vi "host_as ETH hub.vi"() -> ()   [LabVIEW 2021]
uses:
  <vilib>/userdefined/High Color/nirio_resource_hc.ctl
  CTL/states.ctl
  classes/P2P from the network/P2P from the network.lvclass
  CTL/user config.ctl
panel:
  out "error out":errorcluster
  out "Enum":T1
  in  "update and start":bool
  in  "num of PDW on fifo before starting secenario":u32
  in  "P2P sample rate":dbl format="%#_6pHz"
  in  "center frequency (Hz)":dbl format="%#_6pHz"
  in  "RF max power":dbl format="%#_gdBm"
  out "pulse transmitted":u32
  out "num of pulses sent to the FPGA":u32
  in  "devicess":T2[](array[typedef])=["IF_transceiver_0", "IF_transceiver_1", "IF_transceiver_2"]
  in  "receiver port":u16=8800
  in  "vst_device":refnum<k15>[](array[refnum])=["VST_5840"]
  out "secnario elapest 2":dbl
  out "dds free":bool[][](array[boolean])=[[TRUE, FALSE, FALSE, FALSE, FALSE, FALSE], [TRUE, FALSE, FALSE, FALSE, FALSE, FALSE], [TRUE, FALSE, FALSE, FALSE, FALSE, FALSE], [TRUE, FALSE, FALSE, FALSE, FALSE, FALSE], [TRUE, FALSE, FALSE, FALSE, FALSE, FALSE], [TRUE, FALSE, FALSE, FALSE, FALSE, FALSE], [TRUE, FALSE, FALSE, FALSE, FALSE, FALSE], [TRUE, FALSE, FALSE, FALSE, FALSE, FALSE], [TRUE, FALSE, FALSE, FALSE, FALSE, FALSE], [TRUE, TRUE, TRUE, TRUE, TRUE, TRUE], [TRUE, TRUE, TRUE, TRUE, TRUE, TRUE], [TRUE, TRUE, TRUE, TRUE, TRUE, TRUE], [TRUE, TRUE, TRUE, TRUE, TRUE, TRUE], [TRUE, TRUE, TRUE, TRUE, TRUE, TRUE], [TRUE, TRUE, TRUE, TRUE, TRUE, TRUE], [TRUE, TRUE, TRUE, TRUE, TRUE, TRUE]]
  # "HW"
  # "RF setup"
  # "Tx state"
  # "Control"
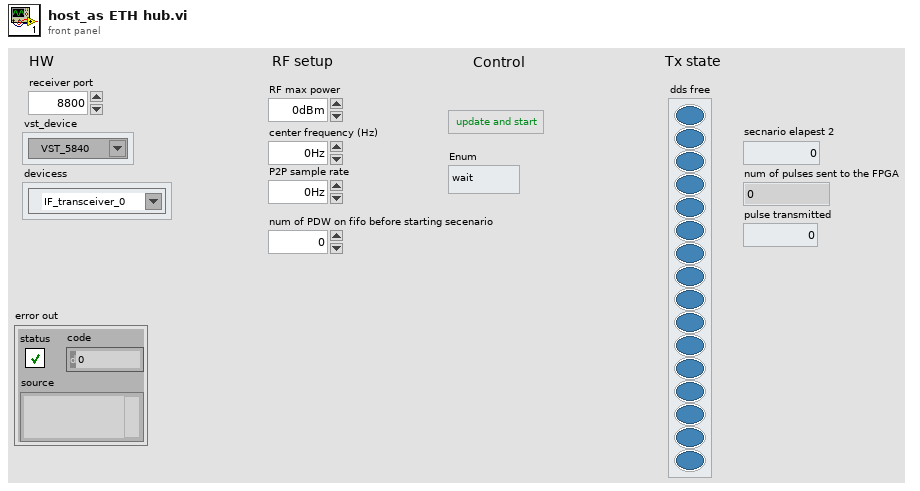
[diagram p1: front panel]
types:
  T1 = typedef "states.ctl" = enum16{"wait", "update config", "ini for transmit", "prime the fifo", "sync and trig", "transmit", "close sesion", "close program", "import secenario from csv", "generate secenario", "refresh file display", "export file", "reset sesion"}
  T2 = typedef "nirio_resource_hc.ctl" = tag
  T3 = typedef "user config.ctl" = cluster{"vst_device":refnum<k15>[], "RF gain ":dbl, "buffer size":u32, "center frequency (Hz) ":dbl, "P2P sample rate":dbl, "mode":enum16{"USRP - 180MHz", "5785 - 2*180MHz", "5785 - 3.2GHz", "P2P - VST"}, "devicess":T2[], "gen for df":bool, "Rx settings":cluster{"min PW         ":dbl, "max gap        ":dbl, "detection bar":dbl, "peak detect                        ":bool}, "IQ file":path}
  T4 = cluster{"fpga clock":dbl, "pulse transmitted":u32, "dds free":bool[][]}
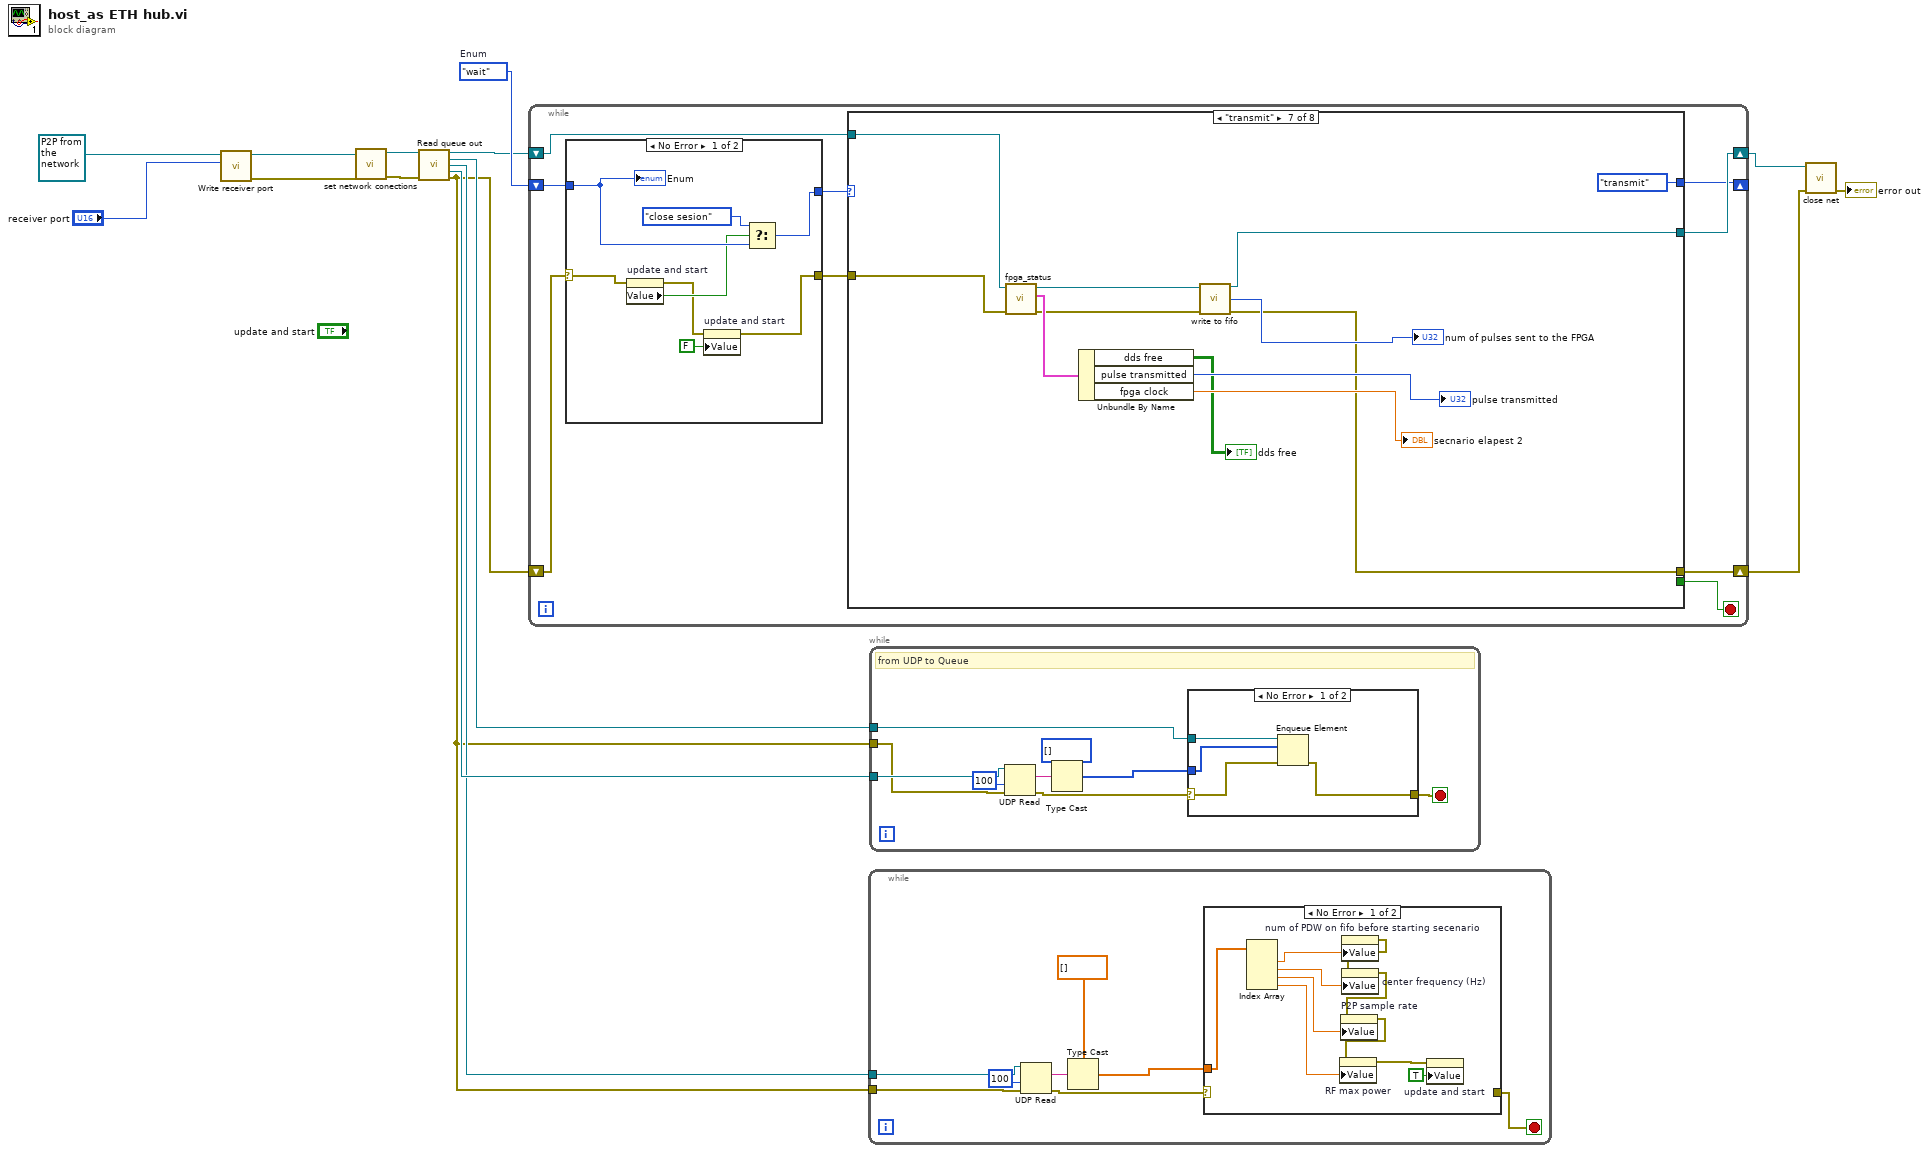
[diagram p0: block diagram]
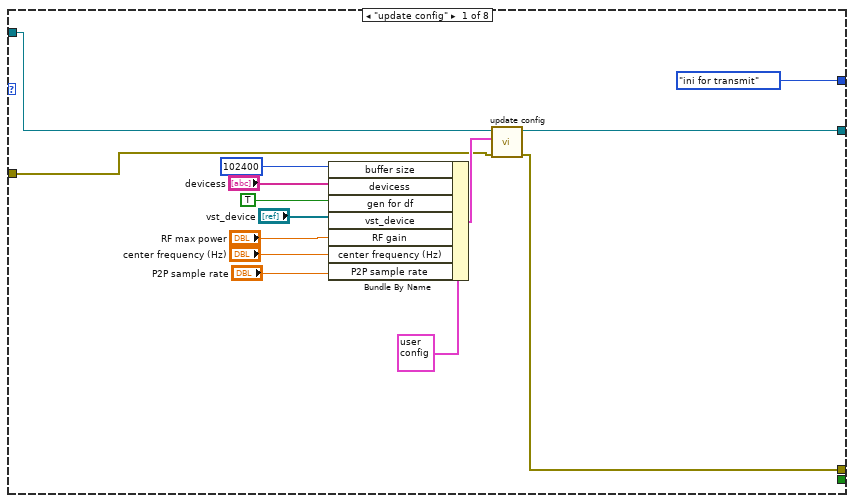
[diagram p2: hidden frame]
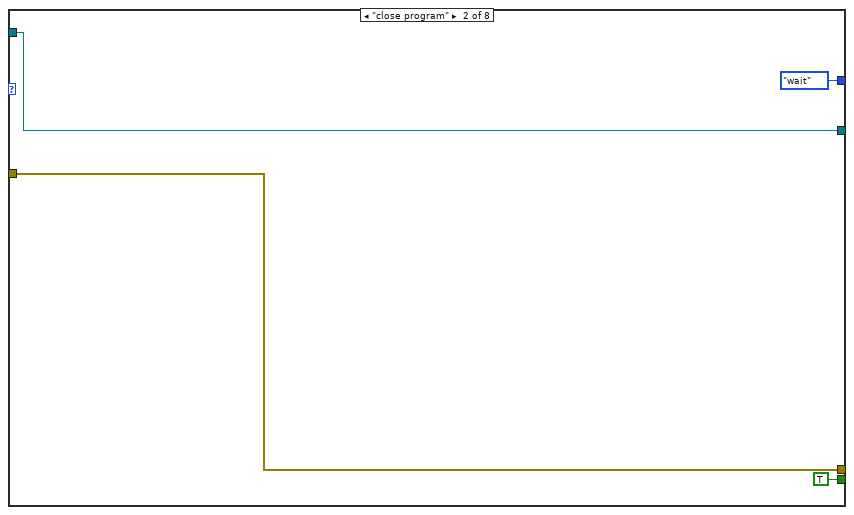
[diagram p3: hidden frame]
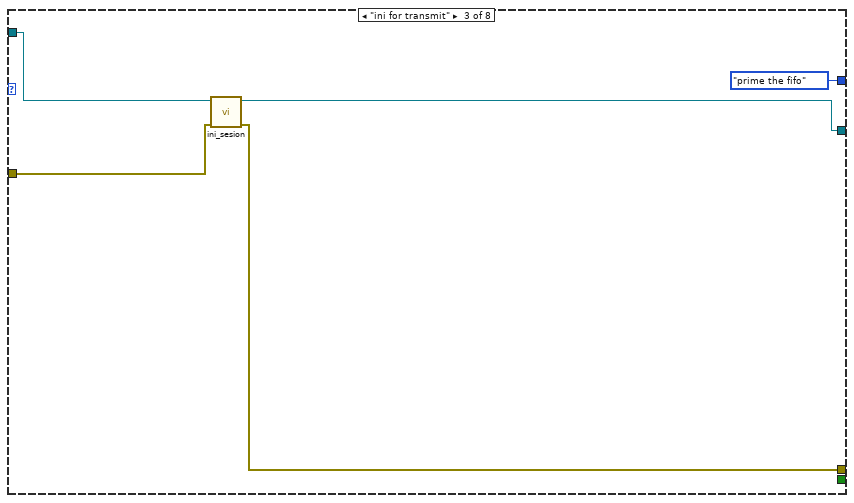
[diagram p4: hidden frame]
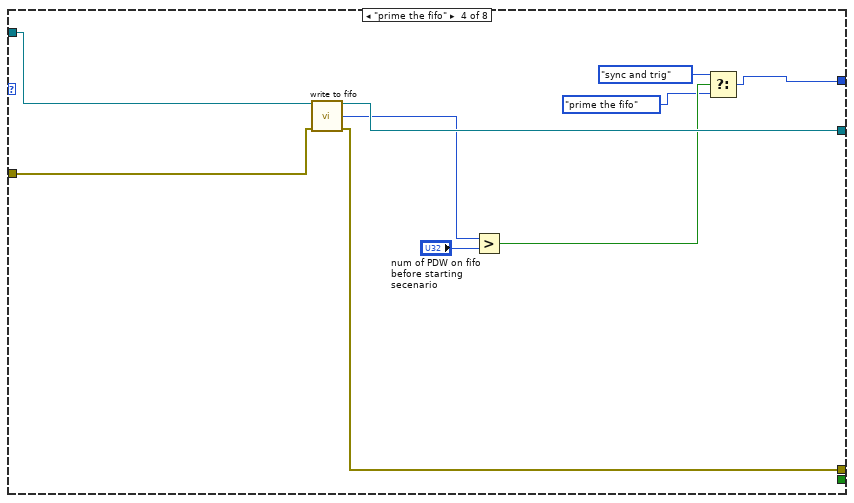
[diagram p5: hidden frame]
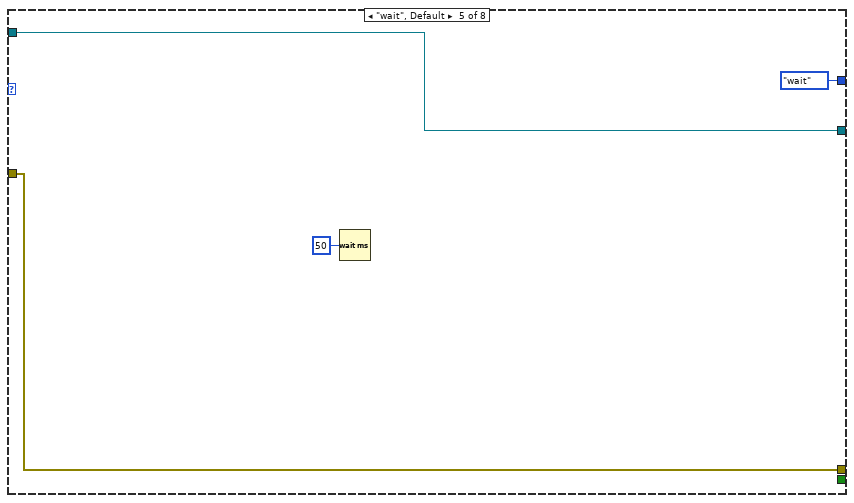
[diagram p6: hidden frame]
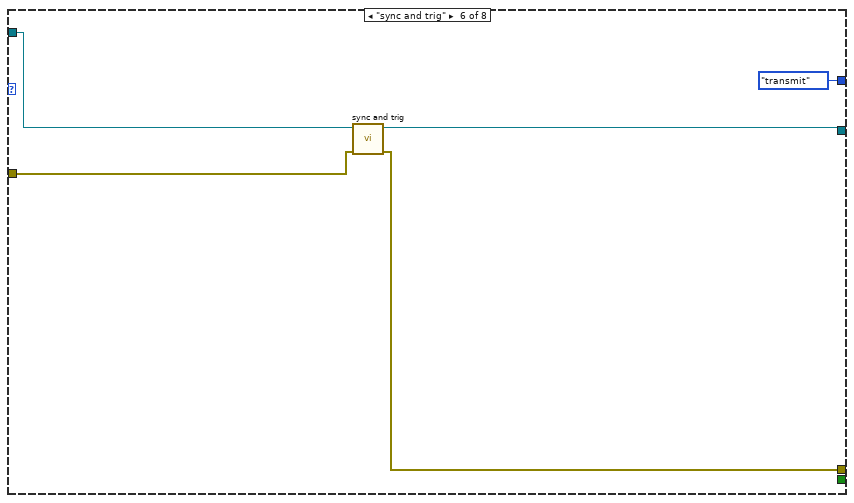
[diagram p7: hidden frame]
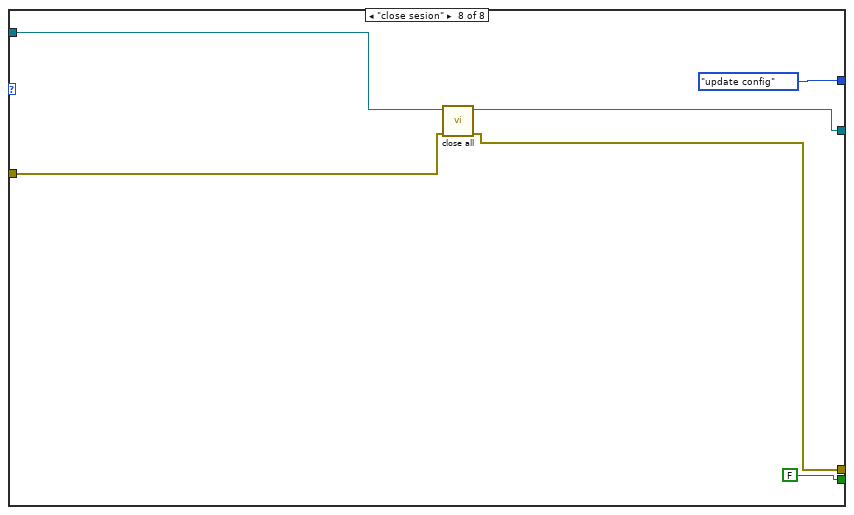
[diagram p8: hidden frame]
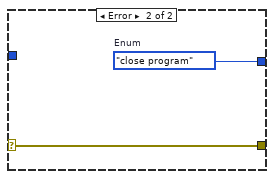
[diagram p9: hidden frame]
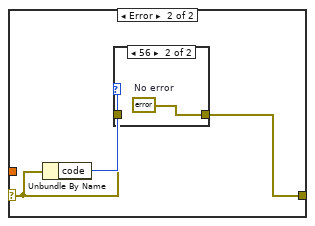
[diagram p10: hidden frame]
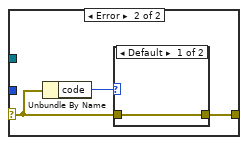
[diagram p12: hidden frame]
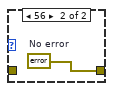
[diagram p13: hidden frame]
diagram:
  w8 = states."wait"  # Enum
  n1 = call-dynamic "Write receiver port.vi"("receiver port"="receiver port", "P2P from the network in"=refnum<class "P2P from the network.lvclass"> refnum ("P2P from the network.lvclass")) -> ("error out"=w10:errorcluster, "P2P from the network out"=w11:refnum<class "P2P from the network.lvclass">)  [unwired: 8 in]
  n2 = call-dynamic "set network conections.vi"("error in (no error)"=w10, "P2P from the network in"=w11) -> ("error out"=w6:errorcluster, "P2P from the network out"=w7:refnum<class "P2P from the network.lvclass">)  [unwired: 8 in]
  n3 = call-dynamic "Read queue out.vi"("P2P from the network in"=w7, "error in (no error)"=w6) -> ("P2P from the network out"=w4:refnum<class "P2P from the network.lvclass">, "queue out"=w14:refnum<queue>, "connection ID control port"=w9:refnum<k16>, "connection ID PDW"=w15:refnum<k16>, "error out"=w5:errorcluster)  [unwired: 9 in]
  n4 = while {
    shift-right: [w16] -> _
    shift-left: w8 -> [w23]
    shift-right: [w18] -> w2
    shift-left: w5 -> [w24]
    shift-right: [w19] -> w3
    shift-left: w4 -> [w21]
    stop <- w17 stop-if-true
    n5 = case shown="No Error" w24 {
      selector: w24 -> [w86 w93]
      tunnel: w23 -> [w92 _]
      tunnel: [w91 w94] -> w22
      tunnel: [w85 w93] -> w20
      frame No Error {
        n6 = property on="update and start" class="Bool (strict)"(error in=w86) -> (error out=w88:errorcluster, "Value"=w89:bool)  [unwired: 1 in, 1 out]
        n7 = property on="update and start" class="Bool (strict)"(error in=w88, "Value"=FALSE ("update and start")) -> (error out=w85:errorcluster)  [unwired: 1 in, 1 out]
        n8 = Select(t=states."close sesion", s=w89, f=w92) -> (s? t:f=w91:T1)
        "Enum" <- w92
      }
      frame Error {
        w94 = states."close program"  # Enum
      }
    }
    n9 = case shown="\"transmit\"" w22 {
      tunnel: w21 -> [w28 w39 w47 w57 w60 w66 w70 w82]
      tunnel: w20 -> [w29 w41 w46 w55 w59 w64 w71 w80]
      tunnel: [w27 w39 w45 w56 w60 w65 w69 w81] -> w19
      tunnel: [states."ini for transmit" ("Enum") states."wait" ("Enum") states."prime the fifo" ("Enum") w49 states."wait" ("Enum") states."transmit" ("Enum") states."transmit" ("Enum") states."update config" ("Enum")] -> w16
      tunnel: [w25 w41 w44 w54 w59 w63 w68 w79] -> w18
      tunnel: [_ TRUE _ _ _ _ _ FALSE] -> w17
      frame "update config" {
        n10 = Bundle By Name(cluster=T3 {"vst_device"=["VST_1", "VST_2"], "RF gain "=10.0, "buffer size"=524288, "center frequency (Hz) "=1000000000.0, "P2P sample rate"=200000000.0, "mode"=enum."5785 - 2*180MHz", "devicess"=["IF_transiver_0", "IF_transiver_1", "IF_transiver_2"], "gen for df"=FALSE, "Rx settings"={"min PW         "=0.0, "max gap        "=0.0, "detection bar"=0.0, "peak detect                        "=FALSE}, "IQ file"=path ""} ("user configurations"), "buffer size"=u32 102400, "devicess"="devicess", "gen for df"=TRUE, "vst_device"="vst_device", "RF gain"="RF max power", "center frequency (Hz)"="center frequency (Hz)", "P2P sample rate"="P2P sample rate") -> (w33:T3)
        n11 = call-dynamic "update config.vi"("error in (no error)"=w29, "user configurations"=w33, "p2p vst in"=w28) -> ("error out"=w25:errorcluster, "p2p vst out"=w27:refnum<class "P2P from the network.lvclass">)  [unwired: 5 in, 2 out]
      }
      frame "close program" {
      }
      frame "ini for transmit" {
        n12 = call-dynamic "ini_sesion.vi"("error in (no error)"=w46, "p2p vst in"=w47) -> ("error out"=w44:errorcluster, "p2p vst out"=w45:refnum<class "P2P from the network.lvclass">)  [unwired: 8 in]
      }
      frame "prime the fifo" {
        n13 = call-dynamic "write to fifo.vi"("P2P from the network in"=w57, "error in (no error)"=w55) -> ("P2P from the network out"=w56:refnum<class "P2P from the network.lvclass">, "num of pulses sent to the FPGA"=w52:u32, "error out"=w54:errorcluster)  [unwired: 9 in, 2 out]
        n14 = Greater?(x=w52, y="num of PDW on fifo before starting secenario") -> (0:w51:bool)
        n15 = Select(t=states."sync and trig", s=w51, f=states."prime the fifo" ("Enum")) -> (s? t:f=w49:T1)
      }
      frame "wait", Default {
        n16 = Wait (ms)(milliseconds to wait=u32 50) -> ()  [unwired: 1 out]
      }
      frame "sync and trig" {
        n17 = call-dynamic "sync and trig.vi"("error in (no error)"=w64, "p2p vst in"=w66) -> ("error out"=w63:errorcluster, "p2p vst out"=w65:refnum<class "P2P from the network.lvclass">)  [unwired: 8 in]
      }
      frame "transmit" {
        n18 = call-dynamic "fpga_status.vi"("error in (no error)"=w71, "p2p vst in"=w70) -> ("error out"=w73:errorcluster, "pulse TX status"=w74:T4, "p2p vst out"=w72:refnum<class "P2P from the network.lvclass">)  [unwired: 7 in]
        n19 = Unbundle By Name(w74) -> ("dds free"=→"dds free":bool[][], "pulse transmitted"=→"pulse transmitted":u32, "fpga clock"=→"secnario elapest 2":dbl)
        n20 = call-dynamic "write to fifo.vi"("P2P from the network in"=w72, "error in (no error)"=w73) -> ("P2P from the network out"=w69:refnum<class "P2P from the network.lvclass">, "num of pulses sent to the FPGA"=→"num of pulses sent to the FPGA":u32, "error out"=w68:errorcluster)  [unwired: 9 in, 2 out]
      }
      frame "close sesion" {
        n21 = call-dynamic "close all.vi"("error in (no error)"=w80, "p2p vst in"=w82) -> ("error out"=w79:errorcluster, "p2p vst out"=w81:refnum<class "P2P from the network.lvclass">)  [unwired: 8 in]
      }
    }
  }
  n22 = while {
    tunnel: w5 -> [w96]
    tunnel: w9 -> [w95]
    stop <- w97 stop-if-true
    n23 = UDP Read(connection ID=w95, timeout ms (25000)=100, 8:w96) -> (data out=w99:string, error out=w102:errorcluster)  [unwired: 4 out]
    n24 = Type Cast(type=dbl[] [], x=w99) -> (*(type *) &x=w101:dbl[])
    n25 = case shown="No Error" w102 {
      selector: w102 -> [_ w114]
      tunnel: [_ w113] -> w97
      tunnel: w101 -> [w112 _]
      frame No Error {
        # "Sender sent data. Update the chart value."
        n26 = Index Array(array=w112) -> (element #1=w108:dbl, element #2=w111:dbl, element #3=w110:dbl, element #4=w109:dbl)  [unwired: 4 in]
        n27 = property on="num of PDW on fifo before starting secenario" class="DigNum (strict)"("Value"=w108) -> (error out=w107:errorcluster)  [unwired: 2 in, 1 out]
        n28 = property on="center frequency (Hz)" class="DigNum (strict)"(error in=w107, "Value"=w111) -> (error out=w106:errorcluster)  [unwired: 1 in, 1 out]
        n29 = property on="P2P sample rate" class="DigNum (strict)"(error in=w106, "Value"=w110) -> (error out=w105:errorcluster)  [unwired: 1 in, 1 out]
        n30 = property on="RF max power" class="DigNum (strict)"(error in=w105, "Value"=w109) -> (error out=w104:errorcluster)  [unwired: 1 in, 1 out]
        n31 = property on="update and start" class="Bool (strict)"(error in=w104, "Value"=TRUE ("update and start")) -> ()  [unwired: 1 in, 2 out]
      }
      frame Error {
        # "Sender did not send data. Ignore timeout error and keep waiting."
        n32 = Unbundle By Name(w114) -> ("code"=w115:i32)
        n33 = case shown="56" w115 {
          tunnel: w114 -> [w116 _]
          tunnel: [w116 w117] -> w113
          frame Default {
          }
          frame 56 {
            w117 = errorcluster {"status"=FALSE, "code"=0, "source"=""}  # No error
          }
        }
      }
    }
  }
  n34 = while {
    tunnel: w5 -> [w122]
    tunnel: w15 -> [w123]
    tunnel: w14 -> [w121]
    stop <- w118 stop-if-true
    # "from UDP to Queue"
    n35 = UDP Read(connection ID=w123, timeout ms (25000)=100, 8:w122) -> (data out=w125:string, error out=w119:errorcluster)  [unwired: 4 out]
    n36 = Type Cast(type=u64[] [], x=w125) -> (*(type *) &x=w120:u64[])
    n37 = case shown="No Error" w119 {
      selector: w119 -> [w128 w132]
      tunnel: [w127 w131] -> w118
      tunnel: w121 -> [w130 _]
      tunnel: w120 -> [w129 _]
      frame No Error {
        # "Sender sent data. Update the chart value."
        n38 = Enqueue Element(queue=w130, element=w129, error in (no error)=w128) -> (error out=w127:errorcluster)  [unwired: 1 in, 2 out]
      }
      frame Error {
        # "Sender did not send data. Ignore timeout error and keep waiting."
        n39 = Unbundle By Name(w132) -> ("code"=w133:i32)
        n40 = case shown="Default" w133 {
          tunnel: w132 -> [w134 _]
          tunnel: [w134 w135] -> w131
          frame Default {
          }
          frame 56 {
            w135 = errorcluster {"status"=FALSE, "code"=0, "source"=""}  # No error
          }
        }
      }
    }
  }
  n41 = call-dynamic "close net.vi"("error in (no error)"=w2, "P2P from the network in"=w3) -> ("error out"=→"error out":errorcluster)  [unwired: 8 in, 1 out]
